vi "CRYAPI TAB MAIN.vi"() -> ()   [LabVIEW 2013]
uses:
  CRYMain Sub Window Global.vi
  DataView/VIEW/CRYNew View Global.vi
  CRYCurveLibrary/Global/CRYCurve Library Global.vi
  user32.dll
panel:
  out "RefSPF":refnum<vi>
  in  "StateOut":bool
  in  "bFitTabControl":bool
  in  "bMouseDown":bool
  in  "bMsg":bool
  in  "bRefresh":bool
  in  "bStop":bool
  in  "bCLOSE_PAGE":bool
  in  "bFLOAT_PAGE":bool
  in  "sData":string
  in  "nData":i32=2
  in  "sMessage":string
  in  "BackVI":refnum<vi>
  in  "WID":i32=2
  in  "bPopMenu":bool
  in  "Tab Control":T1(tab)=enum."***************"
types:
  T1 = enum32{"Data View", "(Step Setup)", "(Project Document)", "(Curves Library)", "(Project)", "(Result View)", "*", "**", "***", "****", "*****", "******", "*******", "********", "*********", "**********", "***********", "************", "*************", "**************", "***************", "15***************", "16****************", "17*****************", "18******************", "19*******************", "20********************", "21*********************", "22**********************", "23***********************", "24************************", "25*************************"}
  T2 = typedef "LVRectTypeDef.ctl" = cluster{"Left":i16, "Top":i16, "Right":i16, "Bottom":i16}
  T3 = typedef "LVPointTypeDef.ctl" = cluster{"Horizontal":i16, "Vertical":i16}
  T4 = typedef "LVBoundsTypeDef.ctl" = cluster{"Width":u32, "Height":u32}
  T5 = typedef "LVPositionTypeDef.ctl" = cluster{"Left":i32, "Top":i32}
  T6 = cluster{"nType":i32, "nParent":i32, "pVIW":refnum<vi>, "pSPW":refnum<vi>, "nTypeF":i32, "pVIF":refnum<vi>, "pSPF":refnum<vi>, "nIDSpliter":i32, "nProperty":i32, "Bound":T2, "nID":i32, "nData":i32, "sData":string, "pWVI":refnum<vi>, "sTitle":string, "cPages":cluster{"nPage":i32, "sTitle":string, "sIcon":string, "pVI":refnum<vi>, "nID":i32}[], "pTab":refnum<vi>, "nIDPages":i32[], "pSPT":refnum<vi>, "sTemp":string, "nDockID":i32, "nDockLR":i32, "sIcon":string}
  T7 = cluster{"nPage":i32, "sTitle":string, "sIcon":string, "pVI":refnum<vi>, "nID":i32}[]
  T8 = cluster{"nPage":i32, "sTitle":string, "sIcon":string, "pVI":refnum<vi>, "nID":i32}
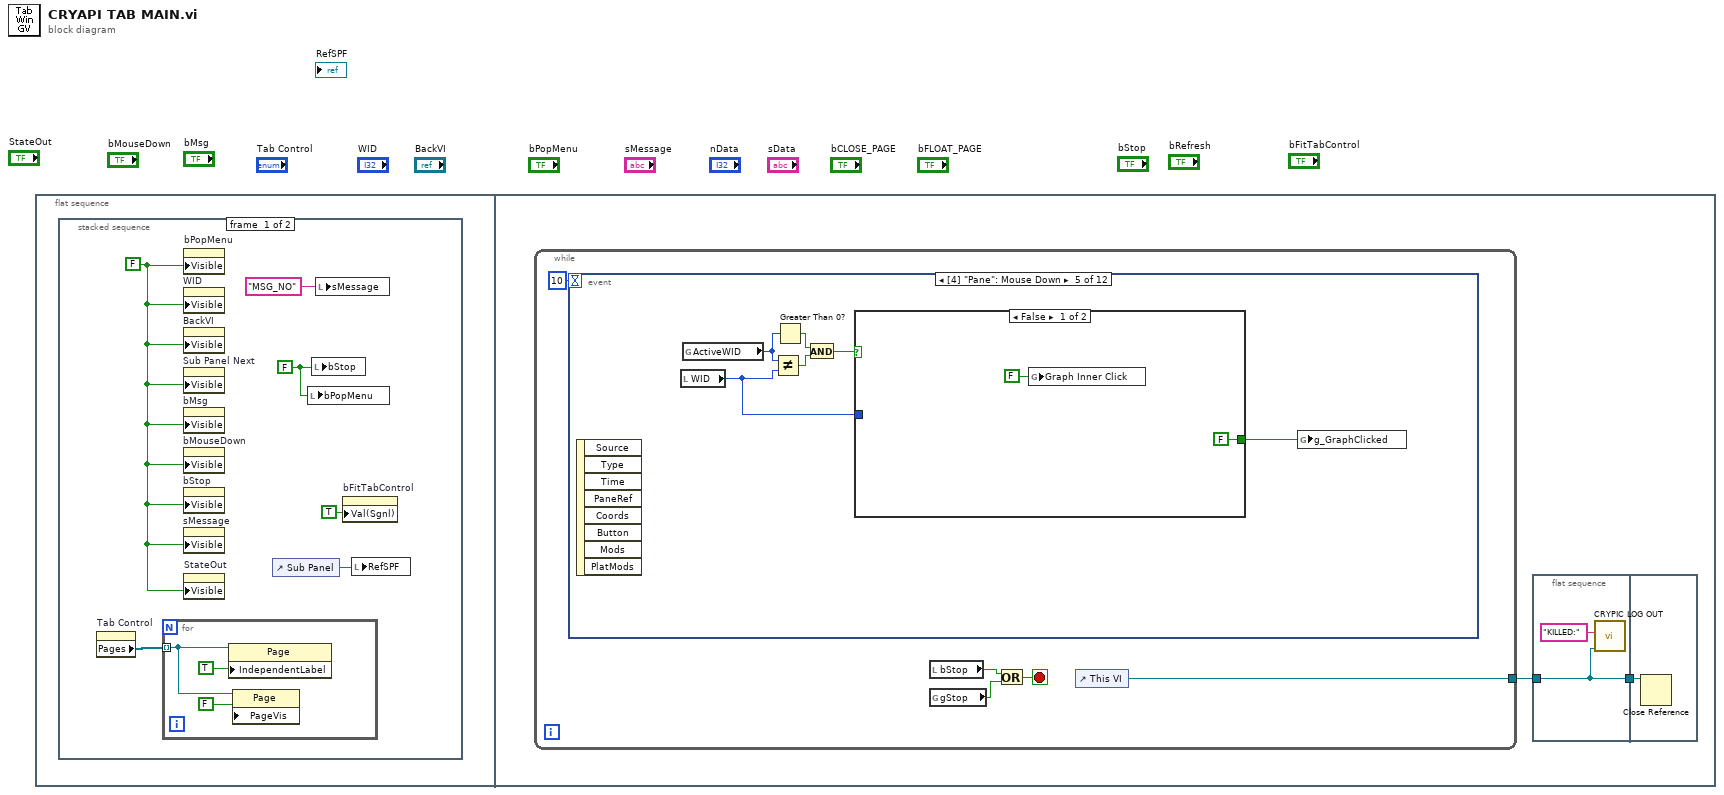
[diagram p0: block diagram]
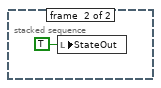
[diagram p2: hidden frame]
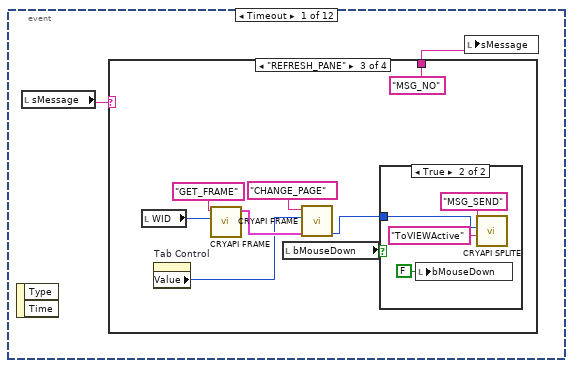
[diagram p3: hidden frame]
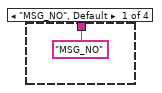
[diagram p4: hidden frame]
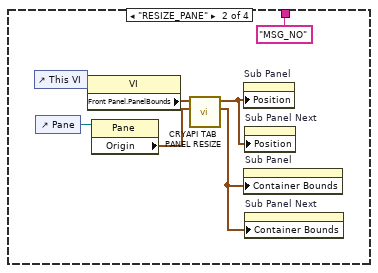
[diagram p5: hidden frame]
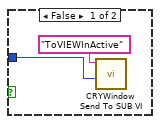
[diagram p6: hidden frame]
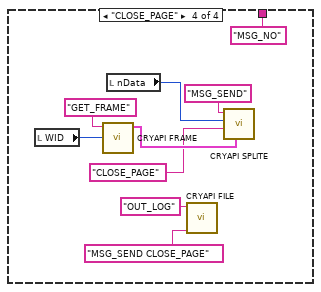
[diagram p7: hidden frame]
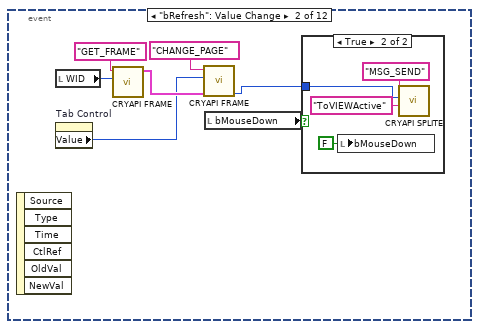
[diagram p8: hidden frame]
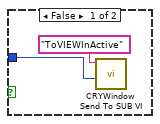
[diagram p9: hidden frame]
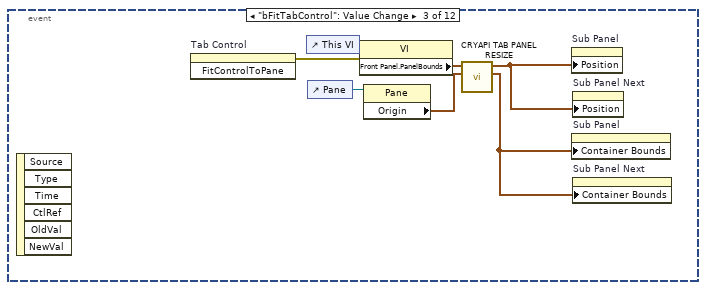
[diagram p10: hidden frame]
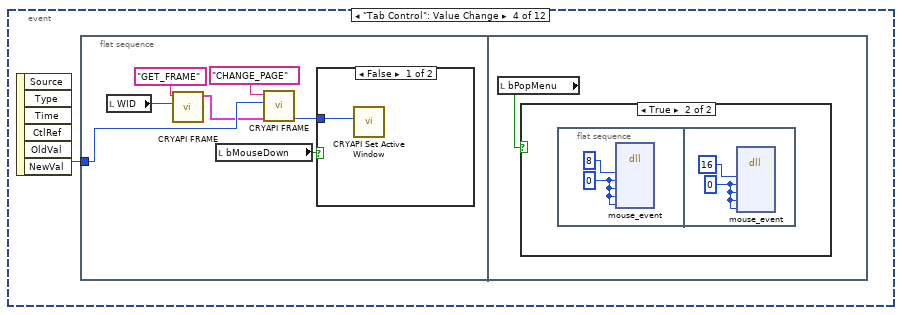
[diagram p11: hidden frame]
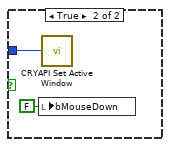
[diagram p12: hidden frame]
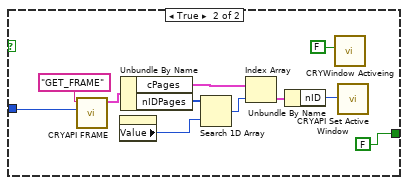
[diagram p14: hidden frame]
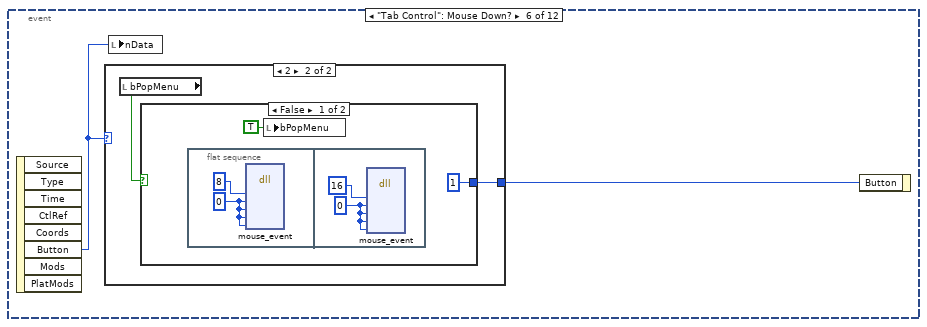
[diagram p15: hidden frame]
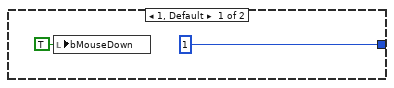
[diagram p16: hidden frame]
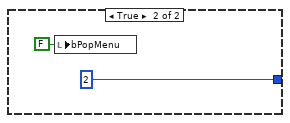
[diagram p17: hidden frame]
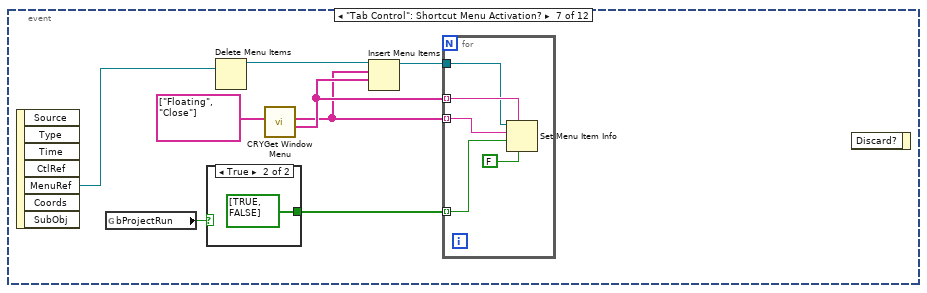
[diagram p18: hidden frame]
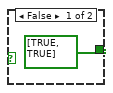
[diagram p19: hidden frame]
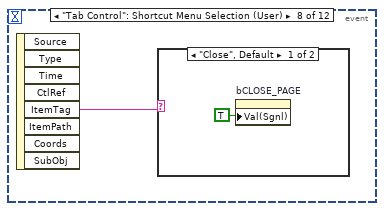
[diagram p20: hidden frame]
diagram:
  n1 = flat-sequence {
    frame #0 {
      n2 = stacked-sequence {
        frame #0 {
          w4 = FALSE ("Visible")
          w2 = FALSE ("Visible")
          n3 = property on="Tab Control" class="TabCtl (strict)"() -> ("Pages"=w6:refnum<vi>[])  [unwired: 2 in, 2 out]
          n4 = for {
            tunnel: w6 -> [w7] mode=indexing
            n5 = property class="Page"(reference=w7, "IndependentLabel"=TRUE ("Independent Label")) -> ()  [unwired: 1 in, 2 out]
            n6 = property class="Page"(reference=w7, "PageVis"=FALSE ("Independent Label")) -> ()  [unwired: 1 in, 2 out]
          }
          n7 = property on="bPopMenu" class="Bool (strict)"("Visible"=w2) -> ()  [unwired: 2 in, 2 out]
          n8 = property on="WID" class="DigNum (strict)"("Visible"=w2) -> ()  [unwired: 2 in, 2 out]
          n9 = property on="BackVI" class="VIRef (strict)"("Visible"=w2) -> ()  [unwired: 2 in, 2 out]
          n10 = property on="Sub Panel Next" class="SubPnl"("Visible"=w2) -> ()  [unwired: 2 in, 2 out]
          n11 = property on="bMsg" class="Bool (strict)"("Visible"=w2) -> ()  [unwired: 2 in, 2 out]
          n12 = property on="bMouseDown" class="Bool (strict)"("Visible"=w2) -> ()  [unwired: 2 in, 2 out]
          n13 = property on="bStop" class="Bool (strict)"("Visible"=w2) -> ()  [unwired: 2 in, 2 out]
          n14 = property on="sMessage" class="Str"("Visible"=w2) -> ()  [unwired: 2 in, 2 out]
          n15 = property on="StateOut" class="Bool (strict)"("Visible"=w2) -> ()  [unwired: 2 in, 2 out]
          n16 = control-ref of="Sub Panel"() -> (w1:refnum<vi>)
          n17 = local write "bPopMenu"(w4) -> ()
          n18 = local write "bStop"(w4) -> ()
          n19 = local write "sMessage"("MSG_NO" ("sMessage")) -> ()
          n20 = property on="bFitTabControl" class="Bool (strict)"("Val(Sgnl)"=TRUE ("Value (Signaling)")) -> ()  [unwired: 2 in, 2 out]
          n21 = local write "RefSPF"(w1) -> ()
        }
        frame #1 {
          n22 = local write "StateOut"(TRUE ("StateOut")) -> ()
        }
      }
    }
    frame #1 {
      n23 = while {
        tunnel: [w19] -> w11
        stop <- w18 stop-if-true
        n24 = event shown="[4] \"Pane\": Mouse Down" {
          selector: _ -> [_ _ _ _ _ _ _ _ _ _ _ _]
          dyn-events: _ -> [_ _ _ _ _ _ _ _ _ _ _ _]
          timeout: 10 -> [_ _ _ _ _ _ _ _ _ _ _ _]
          event Timeout {
            n25 = event-data() -> ()  [unwired: 3 out]
            n26 = local read "sMessage"() -> (w22:string)
            n27 = case shown="\"REFRESH_PANE\"" w22 {
              tunnel: ["MSG_NO" ("sMessage") "MSG_NO" ("sMessage") "MSG_NO" ("sMessage") "MSG_NO" ("sMessage")] -> w21
              frame "MSG_NO", Default {
              }
              frame "RESIZE_PANE" {
                n28 = control-ref of="This VI"() -> (w27:refnum<vi>)
                n29 = control-ref of="Pane"() -> (w28:refnum<vi>)
                n30 = property class="VI"(reference=w27) -> ("Front Panel.PanelBounds"=w29:T2)  [unwired: 1 in, 2 out]
                n31 = property class="Pane"(reference=w28) -> ("Origin"=w30:T3)  [unwired: 1 in, 2 out]
                n32 = call "CRYAPI TAB PANEL RESIZE.vi"("Pane Origin"=w30, "Pane Bound"=w29) -> ("SubPanel Container Bound"=w25:T4, "SubPanel Position"=w26:T5)  [unwired: 8 out]
                n33 = property on="Sub Panel" class="SubPnl"("Position"=w26) -> ()  [unwired: 2 in, 2 out]
                n34 = property on="Sub Panel" class="SubPnl"("Container Bounds"=w25) -> ()  [unwired: 2 in, 2 out]
                n35 = property on="Sub Panel Next" class="SubPnl"("Position"=w26) -> ()  [unwired: 2 in, 2 out]
                n36 = property on="Sub Panel Next" class="SubPnl"("Container Bounds"=w25) -> ()  [unwired: 2 in, 2 out]
              }
              frame "REFRESH_PANE" {
                n37 = local read "WID"() -> (w33:i32)
                n38 = property on="Tab Control" class="TabCtl (strict)"() -> ("Value"=w35:T1)  [unwired: 2 in, 2 out]
                n39 = call "CRYAPI FRAME.vi"("nData"=w33, "sAction"="GET_FRAME") -> ("tFrame_Out"=w36:T6)  [unwired: 4 in, 5 out]
                n40 = local read "bMouseDown"() -> (w32:bool)
                n41 = call "CRYAPI FRAME.vi"("tFrame"=w36, "nData"=w35, "sAction"="CHANGE_PAGE") -> ("nData_Out"=w31:i32)  [unwired: 3 in, 5 out]
                n42 = case shown="True" w32 {
                  tunnel: w31 -> [w39 w42]
                  frame False {
                    n43 = call "CRYWindow Send To SUB VI.vi"("nData"=w39, "sAction"="ToVIEWInActive") -> ()  [unwired: 9 in, 1 out]
                  }
                  frame True {
                    n44 = local write "bMouseDown"(FALSE ("bMouseDown")) -> ()
                    n45 = call "CRYAPI SPLITE.vi"("sData"="ToVIEWActive", "nData"=w42, "sAction"="MSG_SEND") -> ()  [unwired: 6 in, 3 out]
                  }
                }
              }
              frame "CLOSE_PAGE" {
                n46 = local read "WID"() -> (w50:i32)
                n47 = call "CRYAPI FRAME.vi"("nData"=w50, "sAction"="GET_FRAME") -> ("tFrame_Out"=w49:T6)  [unwired: 4 in, 5 out]
                n48 = local read "nData"() -> (w47:i32)
                n49 = call "CRYAPI FILE.vi"("sData"="MSG_SEND CLOSE_PAGE", "sAction"="OUT_LOG") -> ()  [unwired: 8 in, 2 out]
                n50 = call "CRYAPI SPLITE.vi"("tFrame"=w49, "sData"="CLOSE_PAGE", "nData"=w47, "sAction"="MSG_SEND") -> ()  [unwired: 2 in, 6 out]
              }
            }
            n51 = local write "sMessage"(w21) -> ()
          }
          event "bRefresh": Value Change {
            n52 = event-data() -> ()  [unwired: 7 out]
            n53 = local read "WID"() -> (w56:i32)
            n54 = property on="Tab Control" class="TabCtl (strict)"() -> ("Value"=w57:T1)  [unwired: 2 in, 2 out]
            n55 = call "CRYAPI FRAME.vi"("nData"=w56, "sAction"="GET_FRAME") -> ("tFrame_Out"=w58:T6)  [unwired: 4 in, 5 out]
            n56 = call "CRYAPI FRAME.vi"("tFrame"=w58, "nData"=w57, "sAction"="CHANGE_PAGE") -> ("nData_Out"=w54:i32)  [unwired: 3 in, 5 out]
            n57 = local read "bMouseDown"() -> (w55:bool)
            n58 = case shown="True" w55 {
              tunnel: w54 -> [w61 w64]
              frame False {
                n59 = call "CRYWindow Send To SUB VI.vi"("nData"=w61, "sAction"="ToVIEWInActive") -> ()  [unwired: 9 in, 1 out]
              }
              frame True {
                n60 = local write "bMouseDown"(FALSE ("bMouseDown")) -> ()
                n61 = call "CRYAPI SPLITE.vi"("sData"="ToVIEWActive", "nData"=w64, "sAction"="MSG_SEND") -> ()  [unwired: 6 in, 3 out]
              }
            }
          }
          event "bFitTabControl": Value Change {
            n62 = event-data() -> ()  [unwired: 7 out]
            n63 = invoke on="Tab Control" class="TabCtl (strict)" method="FitControlToPane"() -> (error out=w67:errorcluster)  [unwired: 3 in, 2 out]
            n64 = control-ref of="This VI"() -> (w70:refnum<vi>)
            n65 = control-ref of="Pane"() -> (w71:refnum<vi>)
            n66 = property class="VI"(reference=w70, error in=w67) -> ("Front Panel.PanelBounds"=w72:T2)  [unwired: 2 out]
            n67 = property class="Pane"(reference=w71) -> ("Origin"=w73:T3)  [unwired: 1 in, 2 out]
            n68 = call "CRYAPI TAB PANEL RESIZE.vi"("Pane Origin"=w73, "Pane Bound"=w72) -> ("SubPanel Container Bound"=w68:T4, "SubPanel Position"=w69:T5)  [unwired: 8 out]
            n69 = property on="Sub Panel" class="SubPnl"("Position"=w69) -> ()  [unwired: 2 in, 2 out]
            n70 = property on="Sub Panel" class="SubPnl"("Container Bounds"=w68) -> ()  [unwired: 2 in, 2 out]
            n71 = property on="Sub Panel Next" class="SubPnl"("Position"=w69) -> ()  [unwired: 2 in, 2 out]
            n72 = property on="Sub Panel Next" class="SubPnl"("Container Bounds"=w68) -> ()  [unwired: 2 in, 2 out]
          }
          event "Tab Control": Value Change {
            n73 = event-data() -> ("NewVal"=w74:T1)  [unwired: 6 out]
            n74 = flat-sequence {
              tunnel: w74 -> [w79]
              frame #0 {
                n75 = local read "WID"() -> (w77:i32)
                n76 = call "CRYAPI FRAME.vi"("nData"=w77, "sAction"="GET_FRAME") -> ("tFrame_Out"=w78:T6)  [unwired: 4 in, 5 out]
                n77 = local read "bMouseDown"() -> (w76:bool)
                n78 = call "CRYAPI FRAME.vi"("tFrame"=w78, "nData"=w79, "sAction"="CHANGE_PAGE") -> ("nData_Out"=w75:i32)  [unwired: 3 in, 5 out]
                n79 = case shown="False" w76 {
                  tunnel: w75 -> [w82 w83]
                  frame False {
                    n80 = call "CRYAPI Set Active Window.vi"("nData"=w82) -> ()  [unwired: 11 in]
                  }
                  frame True {
                    n81 = local write "bMouseDown"(FALSE ("bMouseDown")) -> ()
                    n82 = call "CRYAPI Set Active Window.vi"("nData"=w83) -> ()  [unwired: 11 in]
                  }
                }
              }
              frame #1 {
                n83 = local read "bPopMenu"() -> (w85:bool)
                n84 = case shown="True" w85 {
                  frame False {
                  }
                  frame True {
                    n85 = flat-sequence {
                      frame #0 {
                        w86 = 0 ("dwDx")
                        n86 = dll-call lib="user32.dll" fn="mouse_event"("dwFlags"=8, "dwDx"=w86, "dwDy"=w86, "dwData"=w86, "dwExtrainfo"=w86) -> ()  [unwired: 9 in, 2 out]
                      }
                      frame #1 {
                        w88 = 0 ("dwDx")
                        n87 = dll-call lib="user32.dll" fn="mouse_event"("dwFlags"=16, "dwDx"=w88, "dwDy"=w88, "dwData"=w88, "dwExtrainfo"=w88) -> ()  [unwired: 9 in, 2 out]
                      }
                    }
                  }
                }
              }
            }
          }
          event Mouse Down {
            n88 = event-data() -> ()  [unwired: 9 out]
            n89 = local read "WID"() -> (w91:i32)
            n90 = global read "CRYMain Sub Window Global.vi" "ActiveWID"() -> (w95:i32)
            n91 = Not Equal?(x=w95, y=w91) -> (x != y?=w94:bool)
            n92 = Greater Than 0?(x=w95) -> (x > 0?=w93:bool)
            n93 = And(x=w93, y=w94) -> (x .and. y?=w92:bool)
            n94 = case shown="False" w92 {
              tunnel: w91 -> [_ w100]
              tunnel: [FALSE ("ActiveTF") FALSE ("ActiveTF")] -> w90
              frame False {
                n95 = global write "CRYCurve Library Global.vi" "Graph Inner Click"(FALSE ("Graph Inner Click")) -> ()
              }
              frame True {
                n96 = call "CRYAPI FRAME.vi"("nData"=w100, "sAction"="GET_FRAME") -> ("tFrame_Out"=w103:T6)  [unwired: 4 in, 5 out]
                n97 = property on="Tab Control" class="TabCtl (strict)"() -> ("Value"=w104:T1)  [unwired: 2 in, 2 out]
                n98 = Unbundle By Name(w103) -> ("cPages"=w105:T7, "nIDPages"=w102:i32[])
                n99 = Search 1D Array(1D array=w102, element=w104) -> (index of element=w106:i32)  [unwired: 1 out]
                n100 = Index Array(array=w105, index=w106) -> (element=w107:T8)
                n101 = Unbundle By Name(w107) -> ("nID"=w99:i32)
                n102 = call "CRYWindow Activeing.vi"("ActiveTF"=FALSE) -> ()  [unwired: 11 in]
                n103 = call "CRYAPI Set Active Window.vi"("nData"=w99) -> ()  [unwired: 11 in]
              }
            }
            n104 = global write "CRYNew View Global.vi" "g_GraphClicked"(w90) -> ()
          }
          event "Tab Control": Mouse Down? {
            n105 = event-data() -> ("Button"=w109:u16)  [unwired: 8 out]
            n106 = case shown="2" w109 {
              tunnel: [1 w114] -> w110
              frame 1, Default {
                n107 = local write "bMouseDown"(TRUE ("bMouseDown")) -> ()
              }
              frame 2 {
                n108 = local read "bPopMenu"() -> (w113:bool)
                n109 = case shown="False" w113 {
                  tunnel: [1 2] -> w114
                  frame False {
                    n110 = flat-sequence {
                      frame #0 {
                        w117 = 0 ("dwDx")
                        n111 = dll-call lib="user32.dll" fn="mouse_event"("dwFlags"=8, "dwDx"=w117, "dwDy"=w117, "dwData"=w117, "dwExtrainfo"=w117) -> ()  [unwired: 9 in, 2 out]
                      }
                      frame #1 {
                        w119 = 0 ("dwDx")
                        n112 = dll-call lib="user32.dll" fn="mouse_event"("dwFlags"=16, "dwDx"=w119, "dwDy"=w119, "dwData"=w119, "dwExtrainfo"=w119) -> ()  [unwired: 9 in, 2 out]
                      }
                    }
                    n113 = local write "bPopMenu"(TRUE ("bPopMenu")) -> ()
                  }
                  frame True {
                    n114 = local write "bPopMenu"(FALSE ("bPopMenu")) -> ()
                  }
                }
              }
            }
            n115 = local write "nData"(w109) -> ()
            n116 = event-data("Button"=w110) -> ()  [unwired: 1 in, 1 out]
          }
          event "Tab Control": Shortcut Menu Activation? {
            n117 = event-data() -> ("MenuRef"=w129:refnum<k9>)  [unwired: 7 out]
            n118 = global read "CRYMain Sub Window Global.vi" "bProjectRun"() -> (w127:bool)
            n119 = case shown="True" w127 {
              tunnel: [bool[] [TRUE, TRUE] bool[] [TRUE, FALSE]] -> w126
              frame False {
              }
              frame True {
              }
            }
            n120 = Delete Menu Items(9:w129) -> (3:w130:refnum<k9>)  [unwired: 3 in, 1 out]
            n121 = call "CRYGet Window Menu.vi"("Tags"=string[] ["Floating", "Close"]) -> ("Tags_Out"=w125:string[], "Names_Out"=w124:string[])  [unwired: 8 in, 1 out]
            n122 = Insert Menu Items(7:w125, 8:w124, 9:w130) -> (3:w123:refnum<k9>)  [unwired: 3 in, 2 out]
            n123 = for {
              tunnel: w126 -> [w132] mode=indexing
              tunnel: w125 -> [w135] mode=indexing
              tunnel: w124 -> [w134] mode=indexing
              tunnel: w123 -> [w131]
              n124 = Set Menu Item Info(6:FALSE ("checked"), 7:w135, 9:w132, 10:w134, 11:w131) -> ()  [unwired: 2 in, 2 out]
            }
            n125 = event-data() -> ()  [unwired: 2 in, 1 out]
          }
          event "Tab Control": Shortcut Menu Selection (User) {
            n126 = event-data() -> ("ItemTag"=w138:string)  [unwired: 8 out]
            n127 = case shown="\"Close\", Default" w138 {
              frame "Close", Default {
                n128 = property on="bCLOSE_PAGE" class="Bool (strict)"("Val(Sgnl)"=TRUE ("Value (Signaling)")) -> ()  [unwired: 2 in, 2 out]
              }
              frame "Floating" {
                n129 = property on="bFLOAT_PAGE" class="Bool (strict)"("Val(Sgnl)"=TRUE ("Value (Signaling)")) -> ()  [unwired: 2 in, 2 out]
              }
            }
          }
          event "Tab Control": Mouse Up; "Tab Control": Mouse Leave {
            n130 = event-data() -> ()  [unwired: 5 out]
          }
          event "bFLOAT_PAGE": Value Change {
            n131 = event-data() -> ()  [unwired: 7 out]
            n132 = local read "WID"() -> (w144:i32)
            n133 = call "CRYAPI FRAME.vi"("nData"=w144, "sAction"="GET_FRAME") -> ("tFrame_Out"=w143:T6)  [unwired: 4 in, 5 out]
            n134 = property on="Tab Control" class="TabCtl (strict)"() -> ("Value"=w142:T1)  [unwired: 2 in, 2 out]
            n135 = call "CRYAPI SPLITE.vi"("tFrame"=w143, "sData"="FLOAT_PAGE", "nData"=w142, "sAction"="MSG_SEND") -> ()  [unwired: 2 in, 6 out]
          }
          event "bCLOSE_PAGE": Value Change {
            n136 = event-data() -> ()  [unwired: 7 out]
            n137 = local read "WID"() -> (w150:i32)
            n138 = call "CRYAPI FRAME.vi"("nData"=w150, "sAction"="GET_FRAME") -> ("tFrame_Out"=w149:T6)  [unwired: 4 in, 5 out]
            n139 = property on="Tab Control" class="TabCtl (strict)"() -> ("Value"=w148:T1)  [unwired: 2 in, 2 out]
            n140 = call "CRYAPI SPLITE.vi"("tFrame"=w149, "sData"="CLOSE_PAGE", "nData"=w148, "sAction"="MSG_SEND") -> ()  [unwired: 2 in, 6 out]
          }
          event Pane Size {
            n141 = event-data() -> ()  [unwired: 7 out]
            n142 = property on="bFitTabControl" class="Bool (strict)"("Val(Sgnl)"=TRUE ("Value (Signaling)")) -> ()  [unwired: 2 in, 2 out]
          }
        }
        n143 = local read "bStop"() -> (w16:bool)
        n144 = global read "CRYMain Sub Window Global.vi" "gStop"() -> (w17:bool)
        n145 = Or(x=w16, y=w17) -> (x .or. y?=w18:bool)
        n146 = control-ref of="This VI"() -> (w19:refnum<vi>)
      }
      n147 = flat-sequence {
        tunnel: [w13] -> w12
        tunnel: w11 -> [w13]
        tunnel: w12 -> [w15]
        frame #0 {
          n148 = call "CRYPIC LOG OUT.vi"("pVIRef"=w13, "sData"="KILLED:") -> ()  [unwired: 10 in]
        }
        frame #1 {
          n149 = Close Reference(reference=w15) -> ()  [unwired: 1 in, 1 out]
        }
      }
    }
  }
